vi "testMyNewVI.vi"(8 "error in (no error)":errorcluster, 11 "TestCase in":refnum<class "MyTestCase.lvclass">) -> (0 "error out":errorcluster, 3 "TestCase out":refnum<class "MyTestCase.lvclass">)   [LabVIEW 2010]
uses:
  MyTestCase.lvclass
  MyClass.lvclass
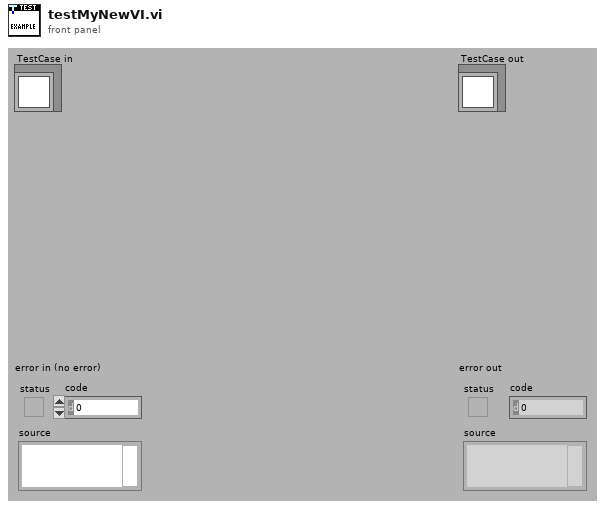
[diagram p1: front panel]
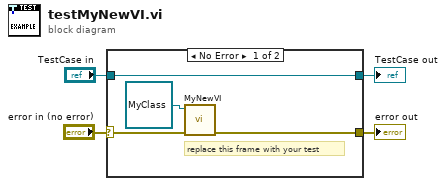
[diagram p0: block diagram]
diagram:
  n1 = case shown="No Error" "error in (no error)" {
    selector: "error in (no error)" -> [w7 w10]
    tunnel: [w6 w10] -> w3
    tunnel: [w8 w9] -> w1
    tunnel: "TestCase in" -> [w8 w9]
    frame No Error {
      # "replace this frame with your test"
      n2 = call-dynamic "MyNewVI.vi"("error in (no error)"=w7, "MyClass in"=refnum<class "MyClass.lvclass"> refnum) -> ("error out"=w6:errorcluster)  [unwired: 8 in, 1 out]
    }
    frame Error {
    }
  }
  "error out" <- w3
  "TestCase out" <- w1
